vi "Set LakeShore 370 Ramp.vi"(8 "error in (no error)":errorcluster, 9 "Ramp rate, K/min":dbl=1.0, 10 "Approach":T1, 11 "VISA resource name":refnum<visa-resource-name>) -> (0 "error out":errorcluster, 3 "VISA resource name out":refnum<visa-resource-name>)   [LabVIEW 2015]
uses:
  Neocera/Neocera Set Point Aproach.ctl
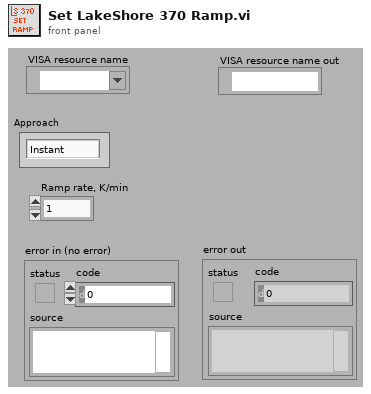
[diagram p1: front panel]
types:
  T1 = typedef "Neocera Set Point Aproach.ctl" = enum16{"Instant", "Ramp"}
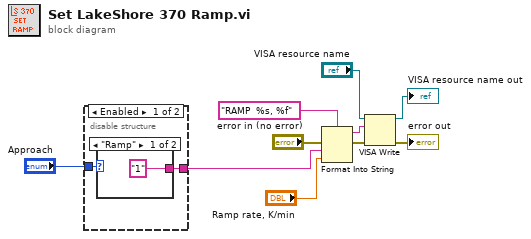
[diagram p0: block diagram]
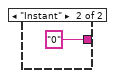
[diagram p2: hidden frame]
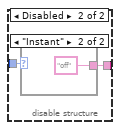
[diagram p3: hidden frame]
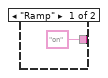
[diagram p4: hidden frame]
diagram:
  n1 = disable-structure shown="Enabled" {
    disable-tunnel: "Approach" -> [w12 w16]
    disable-tunnel: [w11 w15] -> w2
    frame Enabled {
      n2 = case shown="\"Ramp\"" w12 {
        tunnel: ["1" "0"] -> w11
        frame "Ramp" {
        }
        frame "Instant" {
        }
      }
    }
    frame Disabled {
      n3 = case shown="\"Instant\"" w16 {
        tunnel: ["on" "off"] -> w15
        frame "Ramp" {
        }
        frame "Instant" {
        }
      }
    }
  }
  n4 = Format Into String(format string="RAMP  %s, %f" ("write buffer"), error in="error in (no error)", w2, "Ramp rate, K/min") -> (resulting string=w8:string, error out=w9:errorcluster)  [unwired: 1 in]
  n5 = VISA Write(VISA resource name="VISA resource name", write buffer=w8, error in (no error)=w9) -> (VISA resource name out=→"VISA resource name out":refnum<visa-resource-name>, error out=→"error out":errorcluster)  [unwired: 1 out]
